vi "getdata.vi"(7 "condition":bool, 8 "error in (no error)":errorcluster, 10 "inputdata":string, 11 "port":refnum<visa-resource-name>) -> (0 "error out":errorcluster, 1 "VISA resource name":refnum<visa-resource-name>, 2 "end":bool, 3 "outputdata":string)   [LabVIEW 2012]
uses:
  <vilib>/Instr/_visa.llb/VISA Configure Serial Port (Instr).vi
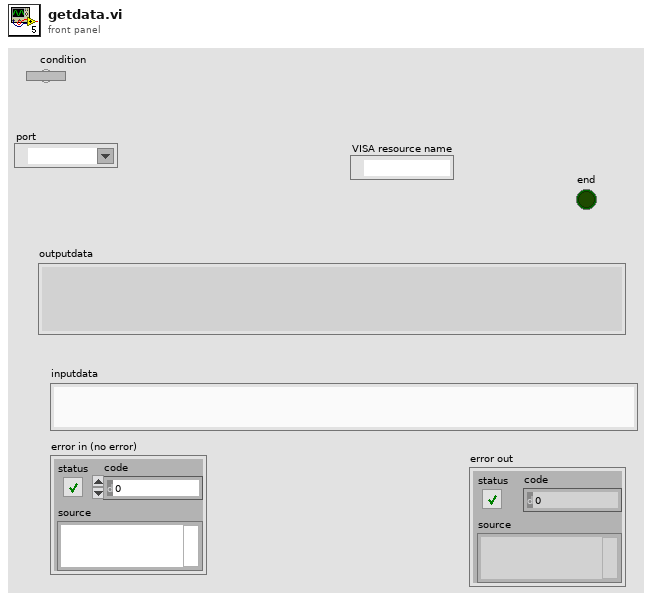
[diagram p1: front panel]
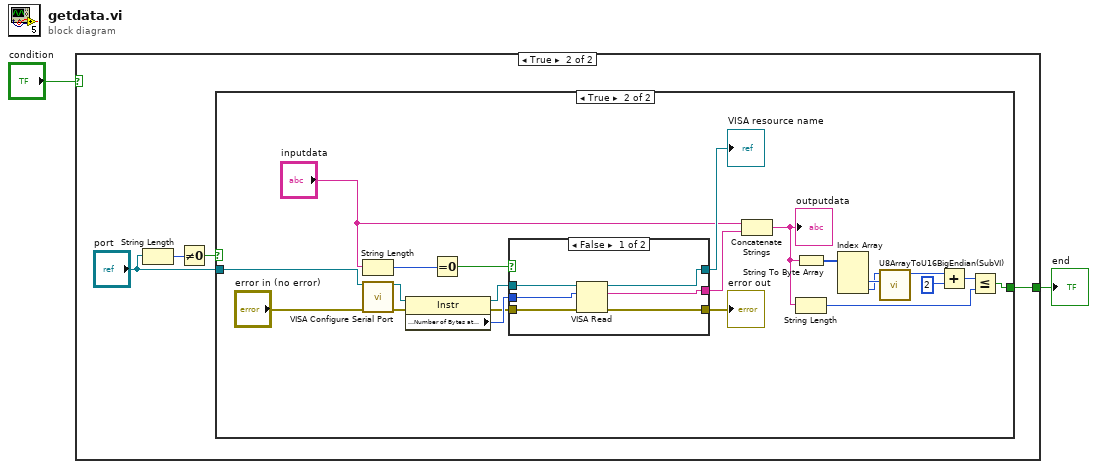
[diagram p0: block diagram]
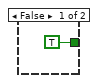
[diagram p2: hidden frame]
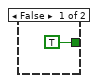
[diagram p3: hidden frame]
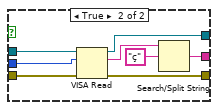
[diagram p4: hidden frame]
diagram:
  n1 = case shown="True" "condition" {
    tunnel: [TRUE w7] -> w2
    frame False {
    }
    frame True {
      n2 = String Length(string="port") -> (length=w6:i32)
      n3 = Not Equal To 0?(x=w6) -> (x != 0?=w5:bool)
      n4 = case shown="True" w5 {
        tunnel: "port" -> [_ w30]
        tunnel: [TRUE w13] -> w7
        frame False {
        }
        frame True {
          n5 = String Length(string="inputdata") -> (length=w21:i32)
          n6 = call-poly "VISA Configure Serial Port"("VISA resource name"=w30, "error in (no error)"="error in (no error)") -> ("VISA resource name out"=w29:refnum<visa-resource-name>, "error out"=w28:errorcluster)  [unwired: 12 in]
          n7 = property class="Instr"(reference=w29, error in=w28) -> (reference out=w18:refnum<visa-resource-name>, error out=w17:errorcluster, "Serial Settings:Number of Bytes at Serial Port"=w19:u32)
          n8 = Equal To 0?(x=w21) -> (x = 0?=w20:bool)
          n9 = case shown="False" w20 {
            tunnel: w19 -> [w34 w44]
            tunnel: w18 -> [w36 w43]
            tunnel: w17 -> [w35 w42]
            tunnel: [w33 w39] -> w16
            tunnel: [w32 w38] -> w11
            tunnel: [w31 w37] -> w10
            frame False {
              n10 = VISA Read(VISA resource name=w36, byte count=w34, error in (no error)=w35) -> (VISA resource name out=w32:refnum<visa-resource-name>, read buffer=w33:string, error out=w31:errorcluster)  [unwired: 1 out]
            }
            frame True {
              n11 = VISA Read(VISA resource name=w43, byte count=w44, error in (no error)=w42) -> (VISA resource name out=w38:refnum<visa-resource-name>, read buffer=w41:string, error out=w37:errorcluster)  [unwired: 1 out]
              n12 = Search/Split String(string=w41, search string/char (-)="ç") -> (match + rest of string=w39:string)  [unwired: 1 in, 2 out]
            }
          }
          "VISA resource name" <- w11
          "error out" <- w10
          n13 = Concatenate Strings("inputdata", w16) -> (w22:string)
          "outputdata" <- w22
          n14 = String To Byte Array(string=w22) -> (unsigned byte array=w27:u8[])
          n15 = String Length(string=w22) -> (length=w14:i32)
          n16 = Index Array(array=w27) -> (element #2=w24:u8, element #3=w23:u8)  [unwired: 3 in, 1 out]
          n17 = call "U8ArrayToU16BigEndian(SubVI).vi"("Numeric 7"=w24, "Numeric 6"=w23) -> ("Numeric 9"=w25:u16)  [unwired: 9 in]
          n18 = Add(x=w25, y=2) -> (x+y=w15:i32)
          n19 = Less Or Equal?(x=w15, y=w14) -> (x <= y?=w13:bool)
        }
      }
    }
  }
  "end" <- w2
